vi "Update_DATA.vi"(8 "error in (no error)":errorcluster, 10 "Name":string, 11 "DATA in":refnum<class "DATA.lvclass">) -> (0 "error out":errorcluster, 3 "DATA out":refnum<class "DATA.lvclass">)   [LabVIEW 2015, in "DATA.lvclass"]
uses:
  DATA.lvclass
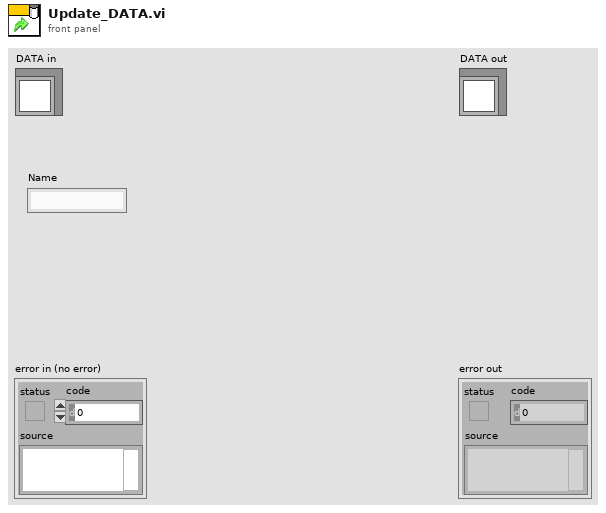
[diagram p1: front panel]
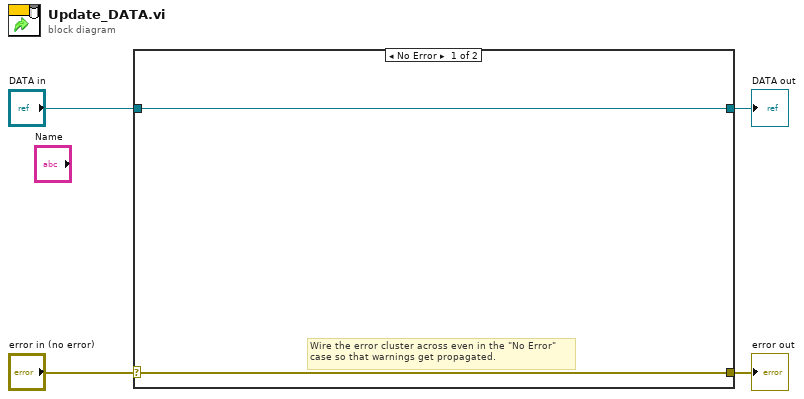
[diagram p0: block diagram]
diagram:
  n1 = case shown="No Error" "error in (no error)" {
    selector: "error in (no error)" -> [w5 w8]
    tunnel: [w5 w8] -> w3
    tunnel: [w6 w7] -> w1
    tunnel: "DATA in" -> [w6 w7]
    frame No Error {
      # "Wire the error cluster across even in the \"No Error\"\ncase so that warnings get propagated."
    }
    frame Error {
    }
  }
  "error out" <- w3
  "DATA out" <- w1
